vi "Arduino_read_serialport.vi"(8 "error in (no error)":errorcluster, 11 "reference":refnum<visa-resource-name>) -> (0 "error out":errorcluster, 1 "Bytes at Port":u32, 2 "String":string, 3 "VISA resource name out":refnum<visa-resource-name>)   [LabVIEW 2015]
panel:
  out "Serial Settings:Number of Bytes at Serial Port after clear":u32
  out "Serial Settings:Number of Bytes at Serial Port":u32
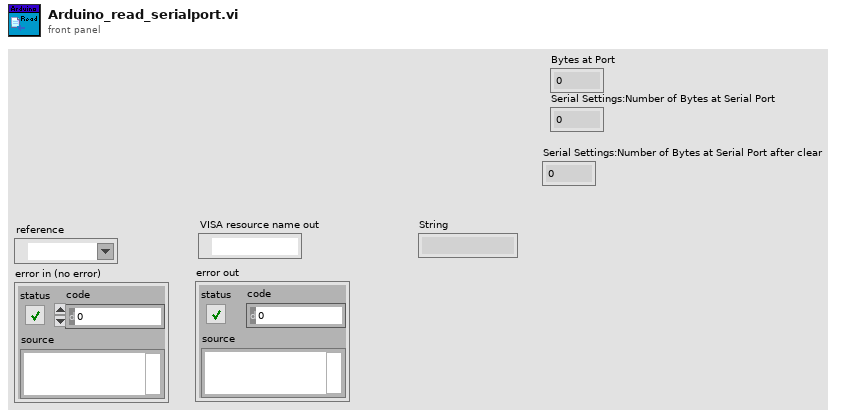
[diagram p1: front panel]
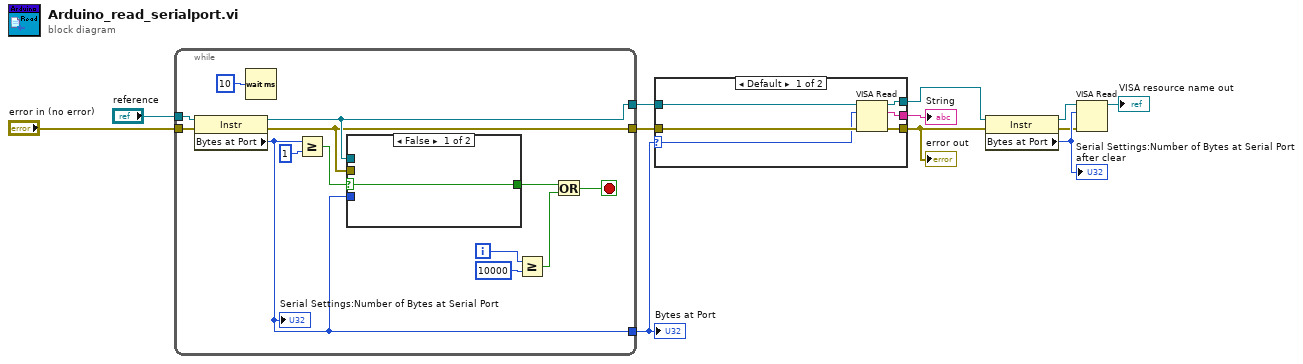
[diagram p0: block diagram]
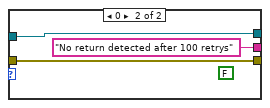
[diagram p2: hidden frame]
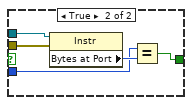
[diagram p3: hidden frame]
diagram:
  n1 = while {
    tunnel: "reference" -> [w24]
    tunnel: "error in (no error)" -> [w23]
    tunnel: [w16] -> w10
    tunnel: [w14] -> w9
    tunnel: [w13] -> w8
    i -> [w22]
    stop <- w18 stop-if-true
    n2 = property class="Instr"(reference=w24, error in=w23) -> (reference out=w14:refnum<visa-resource-name>, error out=w13:errorcluster, "Bytes at Port"=w16:u32)
    "Serial Settings:Number of Bytes at Serial Port" <- w16
    n3 = Wait (ms)(milliseconds to wait=u32 10) -> ()  [unwired: 1 out]
    n4 = Greater Or Equal?(x=w16, y=u32 1) -> (x >= y?=w17:bool)
    n5 = case shown="False" w17 {
      selector: w17 -> [w26 _]
      tunnel: w16 -> [_ w30]
      tunnel: [w26 w29] -> w15
      tunnel: w14 -> [_ w28]
      tunnel: w13 -> [_ w27]
      frame False {
      }
      frame True {
        n6 = property class="Instr"(reference=w28, error in=w27) -> ("Bytes at Port"=w31:u32)  [unwired: 2 out]
        n7 = Equal?(x=w30, y=w31) -> (x = y?=w29:bool)
      }
    }
    n8 = Greater Or Equal?(x=w22, y=10000) -> (x >= y?=w19:bool)
    n9 = Or(x=w15, y=w19) -> (x .or. y?=w18:bool)
  }
  "Bytes at Port" <- w10
  n10 = case shown="Default" w10 {
    selector: w10 -> [w32 _]
    tunnel: [w37 w38] -> w6
    tunnel: [w36 "No return detected after 100 retrys"] -> w7
    tunnel: [w35 w39] -> w5
    tunnel: w9 -> [w34 w39]
    tunnel: w8 -> [w33 w38]
    frame Default {
      n11 = VISA Read(VISA resource name=w34, byte count=w32, error in (no error)=w33) -> (VISA resource name out=w35:refnum<visa-resource-name>, read buffer=w36:string, error out=w37:errorcluster)  [unwired: 1 out]
    }
    frame 0 {
      (unwired) FALSE
    }
  }
  "error out" <- w6
  "String" <- w7
  n12 = property class="Instr"(reference=w5, error in=w6) -> (reference out=w4:refnum<visa-resource-name>, error out=w2:errorcluster, "Bytes at Port"=w3:u32)
  "Serial Settings:Number of Bytes at Serial Port after clear" <- w3
  n13 = VISA Read(VISA resource name=w4, byte count=w3, error in (no error)=w2) -> (VISA resource name out=→"VISA resource name out":refnum<visa-resource-name>)  [unwired: 3 out]
